vi "Initial Data Save first.vi"(8 "error in (no error)":errorcluster, 9 "index":i32=30, 11 "String In":string="$AGENT.81,C8.C8,S*03") -> (0 "error out":errorcluster)   [LabVIEW 2019]
uses:
  Global/Process Global.vi
panel:
  out "機種廠商代號":string
  out "硬體版本":string
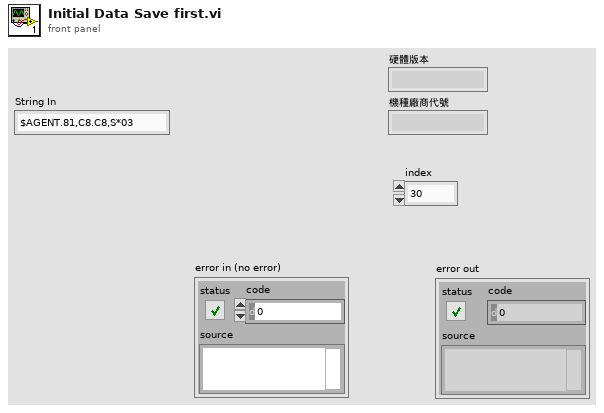
[diagram p1: front panel]
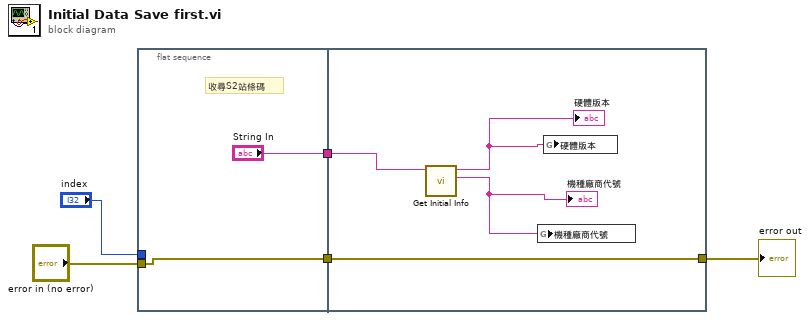
[diagram p0: block diagram]
diagram:
  n1 = flat-sequence {
    tunnel: "error in (no error)" -> [w6]
    tunnel: ["String In"] -> w4
    tunnel: "index" -> [_]
    tunnel: [w6] -> w2
    tunnel: w4 -> [w11]
    tunnel: w2 -> [w8]
    tunnel: [w8] -> w1
    frame #0 {
      # "收尋S2站條碼"
    }
    frame #1 {
      n2 = call "Get Initial Info.vi"("String"=w11) -> ("機種廠商代號"=w10:string, "硬體版本"=w9:string)  [unwired: 9 in]
      "硬體版本" <- w9
      "機種廠商代號" <- w10
      n3 = global write "Process Global.vi" "機種廠商代號"(w10) -> ()
      n4 = global write "Process Global.vi" "硬體版本"(w9) -> ()
    }
  }
  "error out" <- w1
